vi "数据查询_报警信息.vi"() -> ()   [LabVIEW 2016]
uses:
  <vilib>/Utility/miscctls.llb/LVPointTypeDef.ctl
  <vilib>/Utility/miscctls.llb/LVRowAndColumnUnsignedTypeDef.ctl
  <userlib>/_OpenG.lib/array/array.llb/Remove Duplicates from 1D Array (String)__ogtk.vi
  <userlib>/_OpenG.lib/array/array.llb/Sort 2D Array (String)__ogtk.vi
  <vilib>/addons/database/_DB Variant To Data/Database Variant To Data.xnode
panel:
  in  "页":i32 format="第%.0f页"
  in  "每页条数":i32=20
  in  "向后按钮":bool
  in  "向前按钮":bool
  in  "下拉列表":string(xcontrol)
  in  "导出":bool
  in  "查询":bool
  in  "结束日期":string="2050/01/01"
  in  "起始日期":string="2010/01/01"
  out "数据表":string[][](table)
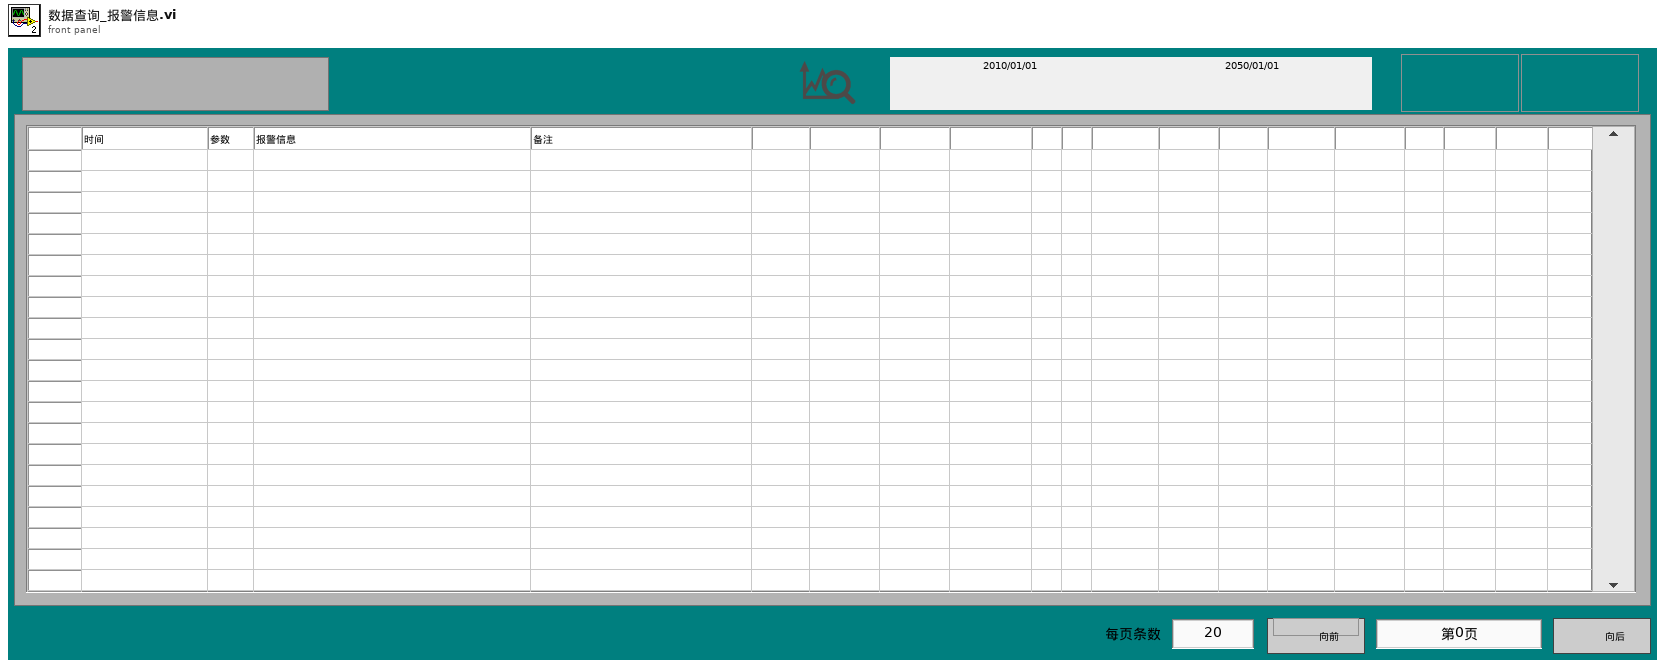
[diagram p1: front panel]
types:
  T1 = typedef "LVPointTypeDef.ctl" = cluster{"Horizontal":i16, "Vertical":i16}
  T2 = typedef "LVDateTimeRec.ctl" = cluster{"秒数的小数部分":dbl, "秒":i32, "分":i32, "时":i32, "日":i32, "月":i32, "年":i32, "天数（周）":i32, "天数（年）":i32, "DST":i32}
  T3 = enum8{"Enabled", "Disabled", "Disabled and Grayed Out"}
  T4 = typedef "LVRowAndColumnUnsignedTypeDef.ctl" = cluster{"Row":u32, "Column":u32}
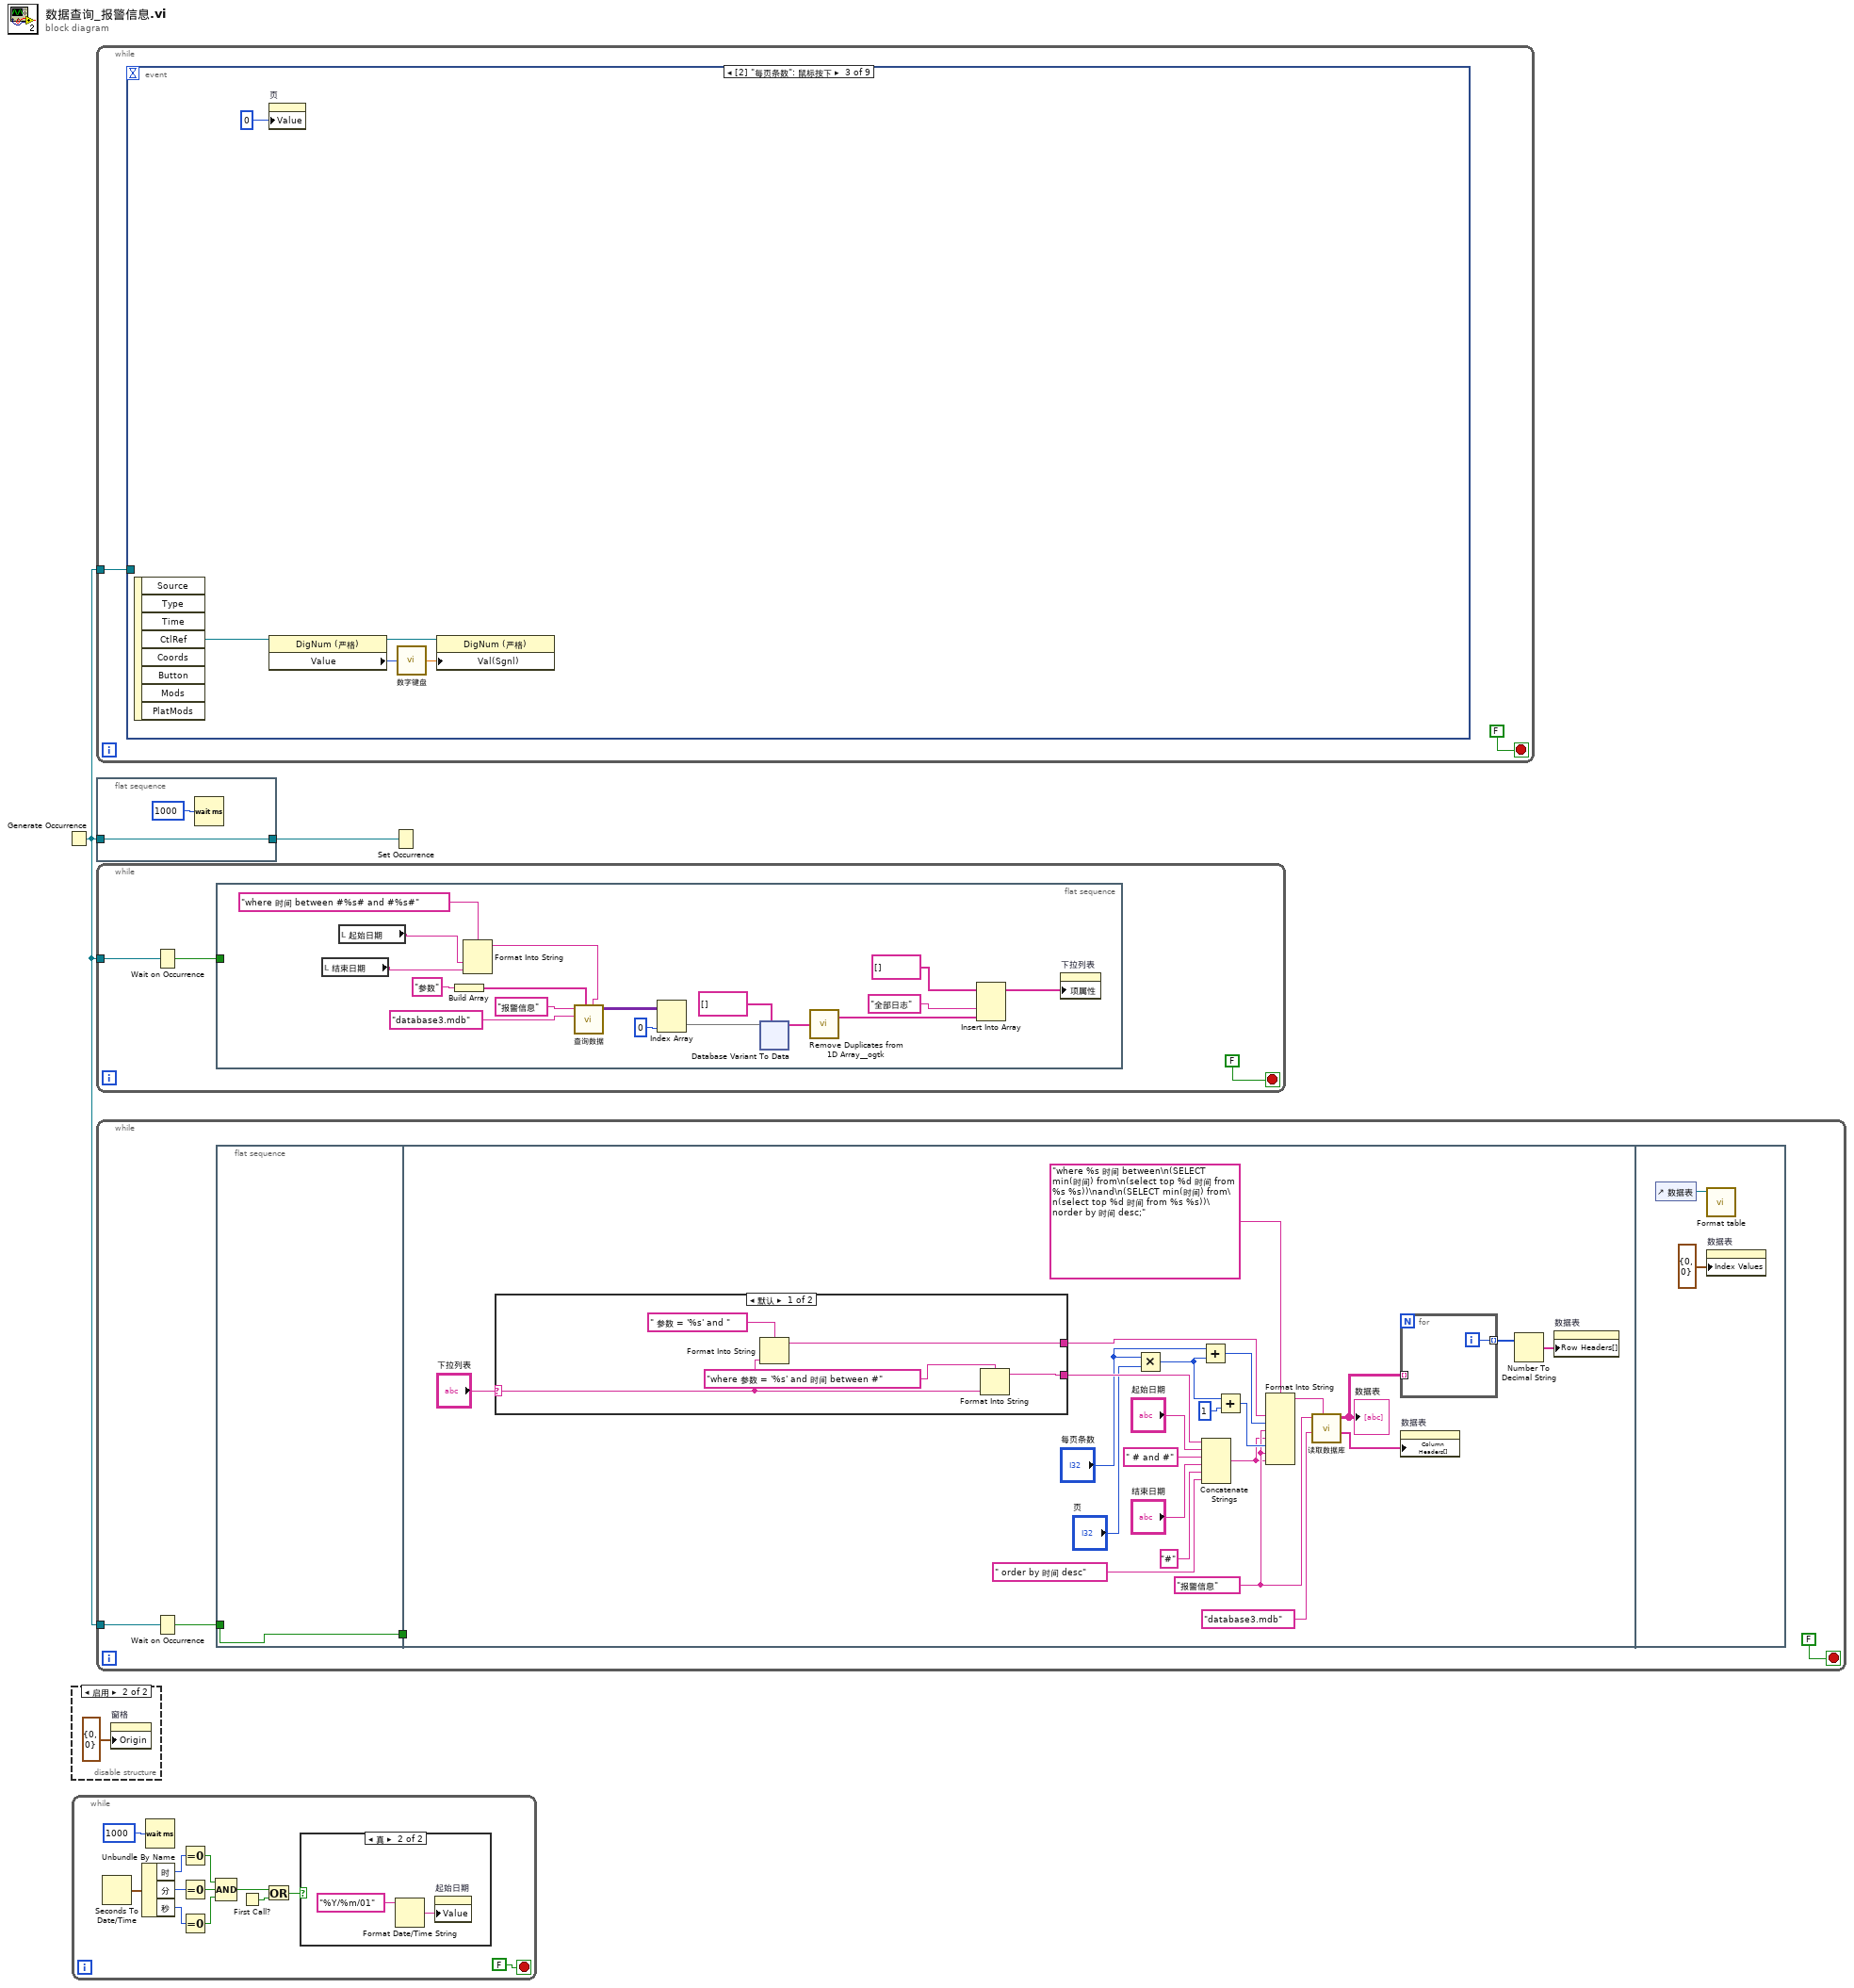
[diagram p0: block diagram]
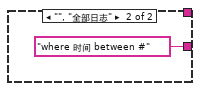
[diagram p2: hidden frame]
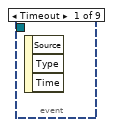
[diagram p4: hidden frame]
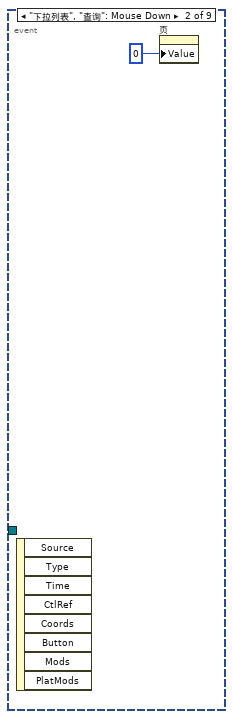
[diagram p5: hidden frame]
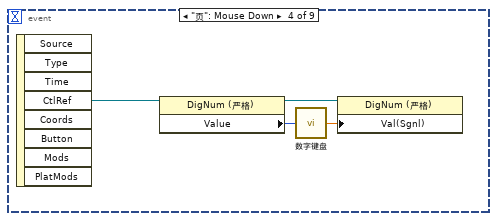
[diagram p6: hidden frame]
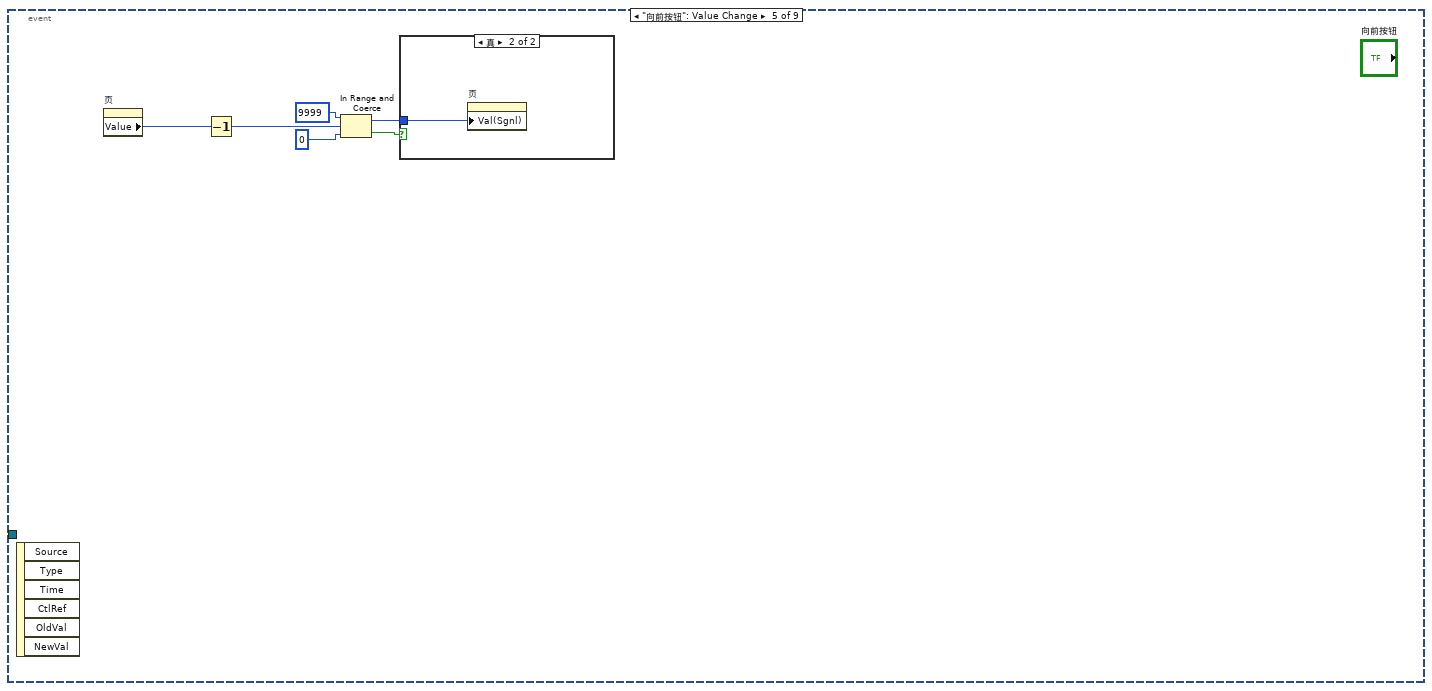
[diagram p7: hidden frame]
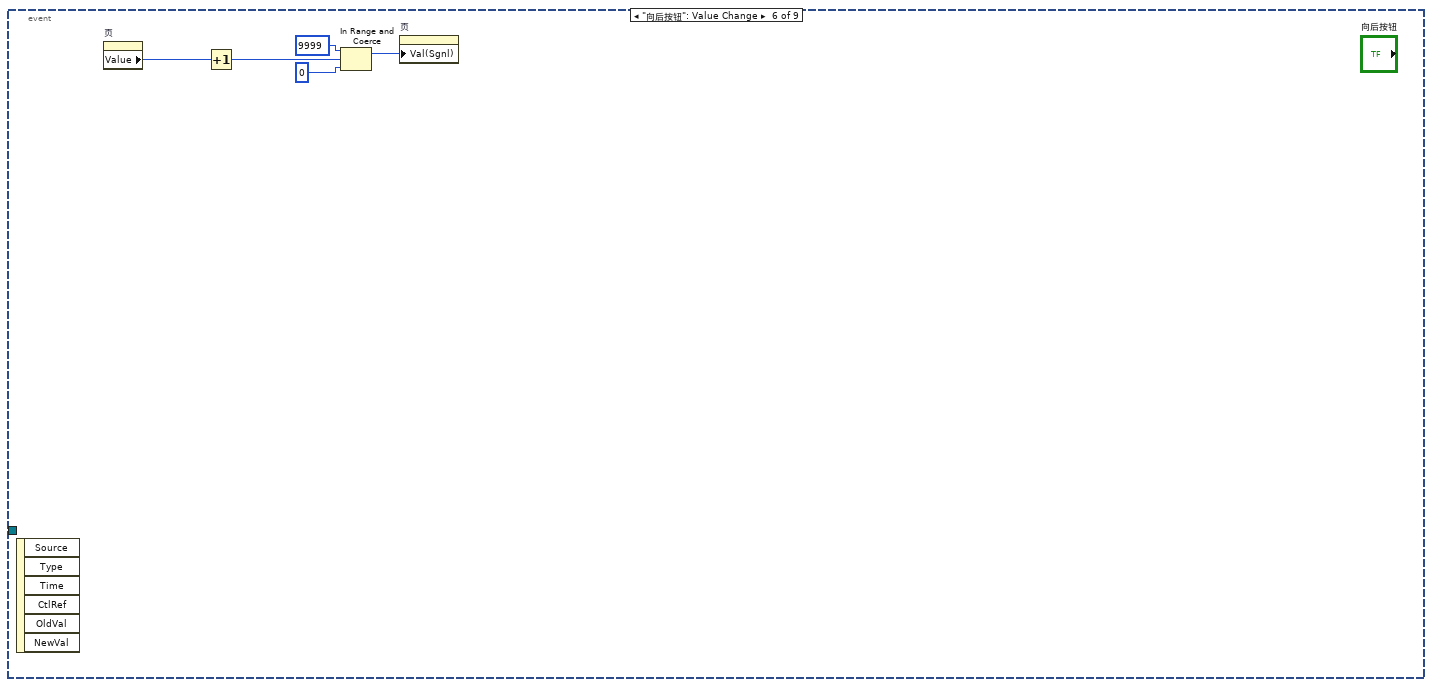
[diagram p9: hidden frame]
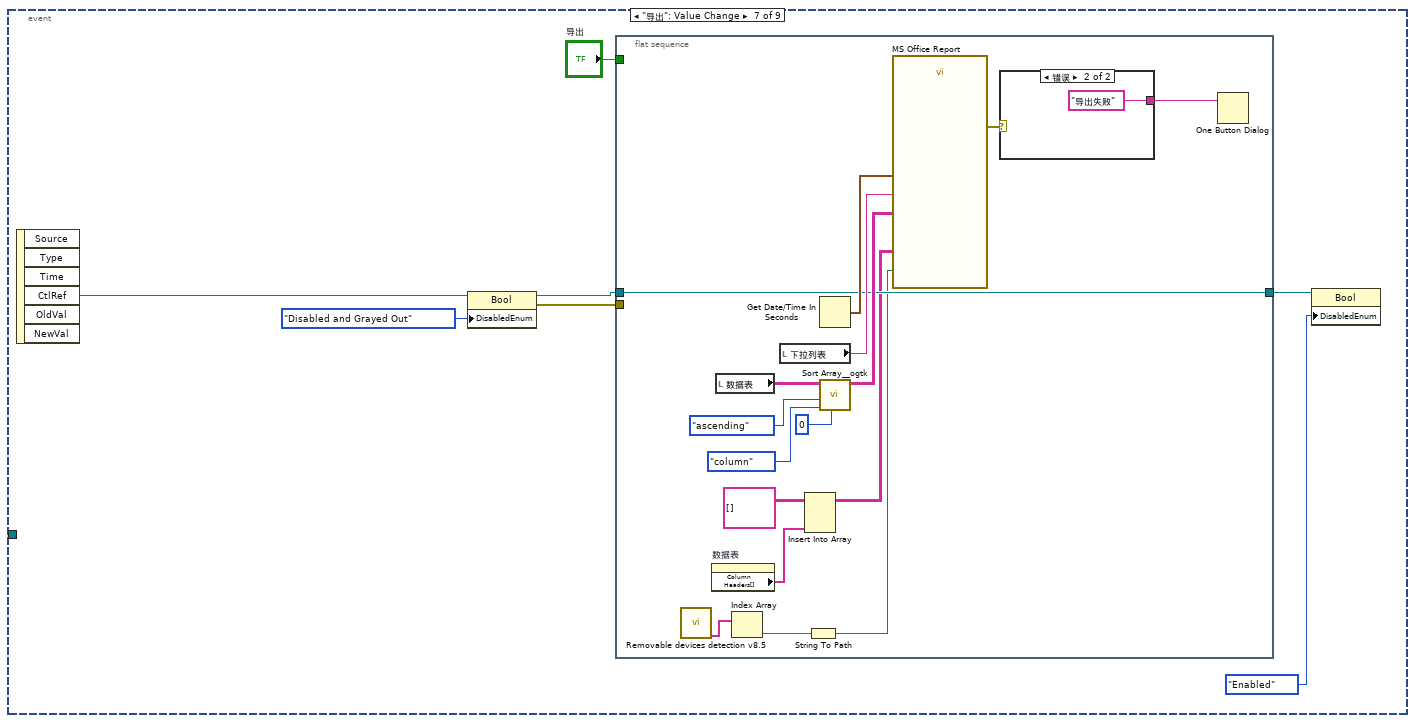
[diagram p10: hidden frame]
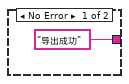
[diagram p11: hidden frame]
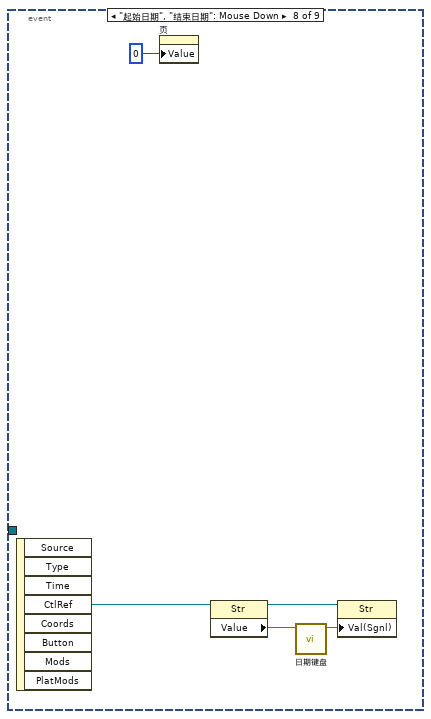
[diagram p12: hidden frame]
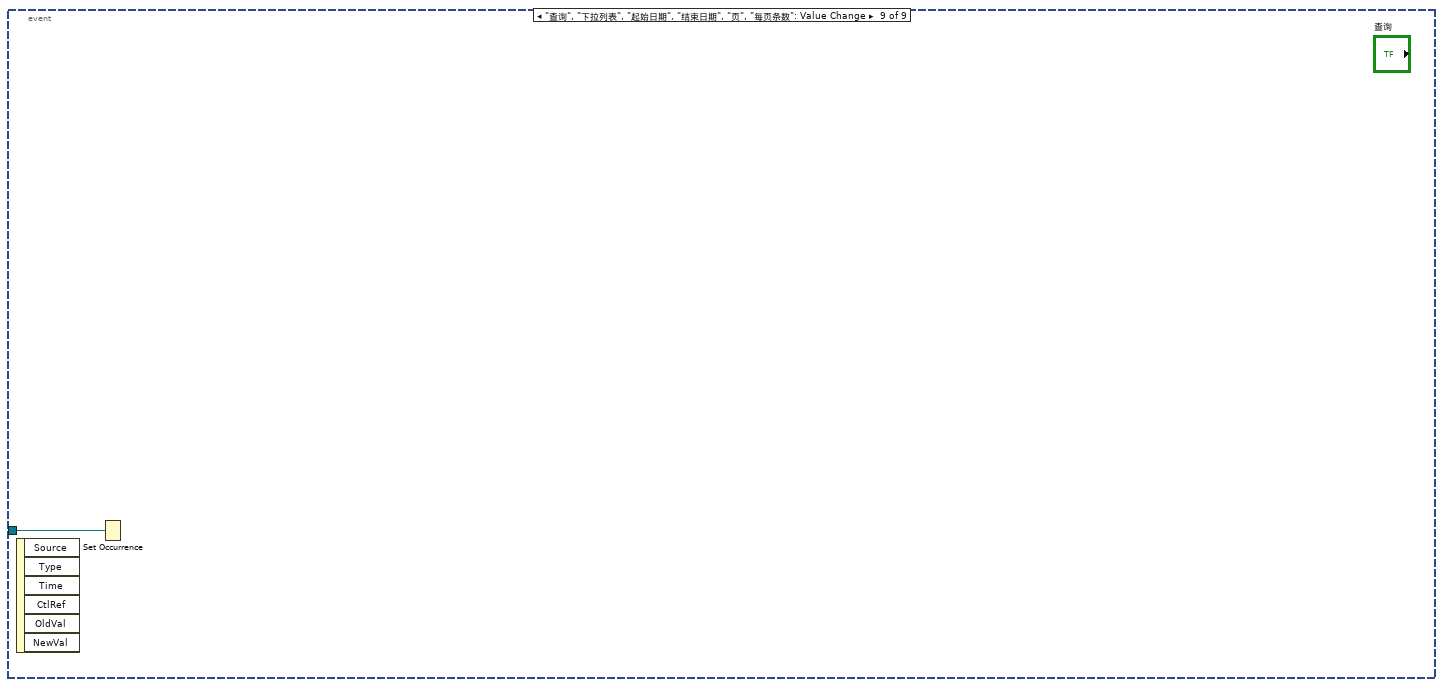
[diagram p13: hidden frame]
diagram:
  n1 = Generate Occurrence() -> (w1:refnum<k4>)
  n2 = disable-structure shown="启用" {
    frame Disabled {
    }
    frame Enabled {
      n3 = property on="窗格" class="Pane"("Origin"=T1 {"Horizontal"=0, "Vertical"=0} ("原点")) -> ()  [unwired: 2 in, 2 out]
    }
  }
  n4 = while {
    stop <- FALSE stop-if-true
    n5 = Seconds To Date/Time() -> (date time rec=w15:T2)  [unwired: 2 in]
    n6 = Unbundle By Name(w15) -> ("时"=w14:i32, "分"=w13:i32, "秒"=w12:i32)
    n7 = Wait (ms)(milliseconds to wait=u32 1000 ("等待时间（毫秒）")) -> ()  [unwired: 1 out]
    n8 = Equal To 0?(x=w14) -> (x = 0?=w11:bool)
    n9 = Equal To 0?(x=w13) -> (x = 0?=w10:bool)
    n10 = Equal To 0?(x=w12) -> (x = 0?=w9:bool)
    n11 = Compound Arithmetic op=AND ("复合运算")(w11, w10, w9) -> (w6:bool)
    n12 = First Call?() -> (First Call?: T/F=w4:bool)
    n13 = Or(x=w6, y=w4) -> (x .or. y?=w5:bool)
    n14 = case shown="真" w5 {
      frame False {
      }
      frame True {
        n15 = Format Date/Time String(time format string (%c)="%Y/%m/01" ("时间格式字符串(%c)")) -> (date/time string=w16:string)  [unwired: 2 in]
        n16 = property on="起始日期" class="Str"("Value"=w16) -> ()  [unwired: 2 in, 2 out]
      }
    }
  }
  n17 = while {
    tunnel: w1 -> [w18]
    stop <- FALSE stop-if-true
    n18 = event shown="[2] \"每页条数\": 鼠标按下" {
      selector: _ -> [_ _ _ _ _ _ _ _ _]
      dyn-events: _ -> [_ _ _ _ _ _ _ _ _]
      timeout: _ -> [_ _ _ _ _ _ _ _ _]
      tunnel: w18 -> [_ _ _ _ _ _ _ _ w72]
      event Timeout {
        n19 = event-data() -> ()  [unwired: 1 in, 3 out]
      }
      event "下拉列表", "查询": Mouse Down {
        n20 = event-data() -> ()  [unwired: 1 in, 8 out]
        n21 = property on="页" class="DigNum (严格)"("Value"=0 ("页")) -> ()  [unwired: 2 in, 2 out]
      }
      event "每页条数": Mouse Down {
        n22 = event-data() -> ("CtlRef"=w22:refnum<vi>)  [unwired: 1 in, 7 out]
        n23 = property on="页" class="DigNum (严格)"("Value"=0 ("页")) -> ()  [unwired: 2 in, 2 out]
        n24 = property class="DigNum (严格)"(reference=w22) -> (reference out=w23:refnum<vi>, "Value"=w25:i32)  [unwired: 1 in, 1 out]
        n25 = call "数字键盘.vi"("OldNumber"=w25) -> ("NewNumber"=w24:dbl)
        n26 = property class="DigNum (严格)"(reference=w23, "Val(Sgnl)"=w24) -> ()  [unwired: 1 in, 2 out]
      }
      event "页": Mouse Down {
        n27 = event-data() -> ("CtlRef"=w26:refnum<vi>)  [unwired: 1 in, 7 out]
        n28 = property class="DigNum (严格)"(reference=w26) -> (reference out=w27:refnum<vi>, "Value"=w29:i32)  [unwired: 1 in, 1 out]
        n29 = call "数字键盘.vi"("OldNumber"=w29) -> ("NewNumber"=w28:dbl)
        n30 = property class="DigNum (严格)"(reference=w27, "Val(Sgnl)"=w28) -> ()  [unwired: 1 in, 2 out]
      }
      event "向前按钮": Value Change {
        n31 = event-data() -> ()  [unwired: 1 in, 6 out]
        n32 = property on="页" class="DigNum (严格)"() -> ("Value"=w35:i32)  [unwired: 2 in, 2 out]
        n33 = Decrement(x=w35) -> (x-1=w34:i32)
        n34 = In Range and Coerce(upper limit=9999 ("上限"), x=w34, lower limit=0 ("下限")) -> (coerced(x)=w31:i32, In Range?=w30:bool)
        n35 = case shown="真" w30 {
          tunnel: w31 -> [_ w36]
          frame False {
          }
          frame True {
            n36 = property on="页" class="DigNum (严格)"("Val(Sgnl)"=w36) -> ()  [unwired: 2 in, 2 out]
          }
        }
      }
      event "向后按钮": Value Change {
        n37 = event-data() -> ()  [unwired: 1 in, 6 out]
        n38 = property on="页" class="DigNum (严格)"() -> ("Value"=w41:i32)  [unwired: 2 in, 2 out]
        n39 = Increment(x=w41) -> (x+1=w40:i32)
        n40 = In Range and Coerce(upper limit=u32 9999 ("上限"), x=w40, lower limit=u32 0 ("下限")) -> (coerced(x)=w37:u32)  [unwired: 1 out]
        n41 = property on="页" class="DigNum (严格)"("Val(Sgnl)"=w37) -> ()  [unwired: 2 in, 2 out]
      }
      event "导出": Value Change {
        n42 = event-data() -> ("CtlRef"=w42:refnum<vi>)  [unwired: 1 in, 5 out]
        n43 = property class="Bool"(reference=w42, "DisabledEnum"=T3."Disabled and Grayed Out" ("禁用")) -> (reference out=w46:refnum<vi>, error out=w47:errorcluster)  [unwired: 1 in]
        n44 = flat-sequence {
          tunnel: w47 -> [_]
          tunnel: [w57] -> w45
          tunnel: w46 -> [w57]
          tunnel: "导出" -> [_]
          frame #0 {
            n45 = call "Removable devices detection v8.5.vi"() -> ("Removable"=w54:string[])  [unwired: 4 out]
            n46 = property on="数据表" class="Tbl (严格)"() -> ("Column Headers[]"=w50:string[])  [unwired: 2 in, 2 out]
            n47 = local read "数据表"() -> (w63:string[][])
            n48 = Index Array(array=w54) -> (element=w53:string)  [unwired: 1 in]
            n49 = local read "下拉列表"() -> (w58:string)
            n50 = Insert Into Array(array=string[][] [], new element=w50) -> (w49:string[][])  [unwired: 2 in]
            n51 = String To Path(string=w53) -> (path=w52:path)
            n52 = Get Date/Time In Seconds() -> (seconds since 1Jan1904=w64:timestamp)
            n53 = call-poly <userlib>:"Sort Array__ogtk.vi"("Column/Row to Sort By"=u32 0, "Sort By in"=enum16{"row", "column"}."column", "Order"=enum16{"ascending", "descending"}."ascending", "Array in"=w63) -> ("Sorted Array out"=w62:string[][])  [unwired: 4 in, 3 out]
            n54 = call "MS Office Report"("Path to Save Report"=w52, "导出日期"=w64, "监测参数"=w58, "数据输入"=w62, "字段定义"=w49) -> ("error out"=w56:errorcluster)  [unwired: 21 in, 1 out]
            n55 = case shown="错误" w56 {
              tunnel: ["导出成功" ("消息") "导出失败" ("消息")] -> w55
              frame No Error {
              }
              frame Error {
              }
            }
            n56 = One Button Dialog(message=w55) -> ()  [unwired: 1 in, 1 out]
          }
        }
        n57 = property class="Bool"(reference=w45, "DisabledEnum"=T3."Enabled" ("禁用")) -> ()  [unwired: 1 in, 2 out]
      }
      event "起始日期", "结束日期": Mouse Down {
        n58 = event-data() -> ("CtlRef"=w71:refnum<vi>)  [unwired: 1 in, 7 out]
        n59 = property on="页" class="DigNum (严格)"("Value"=0 ("页")) -> ()  [unwired: 2 in, 2 out]
        n60 = property class="Str"(reference=w71) -> (reference out=w69:refnum<vi>, "Value"=w70:string)  [unwired: 1 in, 1 out]
        n61 = call "日期键盘.vi"("原值"=w70) -> ("x+y"=w68:string)  [unwired: 10 in]
        n62 = property class="Str"(reference=w69, "Val(Sgnl)"=w68) -> ()  [unwired: 1 in, 2 out]
      }
      event "查询", "下拉列表", "起始日期", "结束日期", "页", "每页条数": Value Change {
        n63 = event-data() -> ()  [unwired: 1 in, 6 out]
        n64 = Set Occurrence(w72) -> ()
      }
    }
  }
  n65 = flat-sequence {
    tunnel: w1 -> [w74]
    tunnel: [w74] -> w2
    frame #0 {
      n66 = Wait (ms)(milliseconds to wait=u32 1000 ("等待时间（毫秒）")) -> ()  [unwired: 1 out]
    }
  }
  n67 = while {
    tunnel: w1 -> [w75]
    stop <- FALSE stop-if-true
    n68 = Wait on Occurrence(2:w75) -> (0:w76:bool)  [unwired: 2 in]
    n69 = flat-sequence {
      tunnel: w76 -> [_]
      frame #0 {
        n70 = local read "结束日期"() -> (w78:string)
        n71 = local read "起始日期"() -> (w79:string)
        n72 = Build Array("参数") -> (w89:string[])
        n73 = Format Into String(format string="where 时间 between #%s# and #%s#" ("格式字符串"), w79, w78) -> (resulting string=w80:string)  [unwired: 2 in, 1 out]
        n74 = call "查询数据.vi"("condition"=w80, "columns"=w89, "database"="database3.mdb", "table"="报警信息") -> ("data"=w88:variant[][])  [unwired: 6 in, 1 out]
        n75 = Index Array(array=w88, index (col)=0 ("禁用的索引 (列)")) -> (element=w87:variant[])  [unwired: 1 in]
        n76 = xnode "Database Variant To Data"("database variant"=w87, "type"=string[] []) -> ("data"=w84:string[])  [unwired: 1 in, 1 out]
        n77 = call-poly <userlib>:"Remove Duplicates from 1D Array__ogtk.vi"("Input Array"=w84) -> ("Output Array"=w83:string[])  [unwired: 1 out]
        n78 = Insert Into Array(array=string[] [], new element #1="全部日志" ("新元素/子数组"), new element #2=w83) -> (w82:string[])  [unwired: 1 in]
        n79 = property on="下拉列表" class="下拉列表 (严格)"("项属性"=w82) -> ()  [unwired: 2 in, 2 out]
      }
    }
  }
  n80 = while {
    tunnel: w1 -> [w135]
    stop <- FALSE stop-if-true
    n81 = Wait on Occurrence(2:w135) -> (0:w134:bool)  [unwired: 2 in]
    n82 = flat-sequence {
      tunnel: w134 -> [w137]
      tunnel: [w137] -> w133
      tunnel: w133 -> [_]
      frame #0 {
      }
      frame #1 {
        w141 = "报警信息" ("组合框")
        n83 = case shown="默认" "下拉列表" {
          selector: "下拉列表" -> [w162 _]
          tunnel: [w165 "where 时间 between #" ("condition")] -> w150
          tunnel: [w161 _] -> w138
          frame Default {
            n84 = Format Into String(format string=" 参数 = '%s' and " ("condition"), w162) -> (resulting string=w161:string)  [unwired: 2 in, 1 out]
            n85 = Format Into String(format string="where 参数 = '%s' and 时间 between #" ("condition"), w162) -> (resulting string=w165:string)  [unwired: 2 in, 1 out]
          }
          frame "", "全部日志" {
          }
        }
        n86 = Multiply(x="每页条数", y="页") -> (x*y=w147:i32)
        n87 = Add(x="每页条数", y=w147) -> (x+y=w145:i32)
        n88 = Concatenate Strings(w150, "起始日期", " # and #" ("condition"), "结束日期", "#" ("condition"), " order by 时间 desc" ("字符串")) -> (w140:string)
        n89 = Add(x=w147, y=u32 1) -> (x+y=w144:u32)
        n90 = Format Into String(format string="where %s 时间 between\n(SELECT min(时间) from\n(select top %d 时间 from %s %s))\nand\n(SELECT min(时间) from\n(select top %d 时间 from %s %s))\norder by 时间 desc;" ("格式字符串"), w138, w145, w141, w140, w144, w141, w140) -> (resulting string=w139:string)  [unwired: 2 in, 1 out]
        n91 = call "读取数据库.vi"("condition"=w139, "database"="database3.mdb", "组合框"=w141) -> ("columns"=w156:string[], "表格"=w154:string[][])  [unwired: 5 in, 2 out]
        "数据表" <- w154
        n92 = for {
          tunnel: w154 -> [_] mode=indexing
          tunnel: [w167] -> w153 mode=indexing
          i -> [w167]
        }
        n93 = property on="数据表" class="Tbl (严格)"("Column Headers[]"=w156) -> ()  [unwired: 2 in, 2 out]
        n94 = Number To Decimal String(number=w153) -> (decimal integer string=w152:string[])  [unwired: 1 in]
        n95 = property on="数据表" class="Tbl (严格)"("Row Headers[]"=w152) -> ()  [unwired: 2 in, 2 out]
      }
      frame #2 {
        n96 = control-ref of="数据表"() -> (w168:refnum<vi>)
        n97 = call "Format table.vi"("Table输入"=w168) -> ()  [unwired: 11 in]
        n98 = property on="数据表" class="Tbl (严格)"("Index Values"=T4 {"Row"=0, "Column"=0} ("索引值")) -> ()  [unwired: 2 in, 2 out]
      }
    }
  }
  n99 = Set Occurrence(w2) -> ()
